vi "Parameter Set Write Single.vi"() -> ()   [LabVIEW 2023, in "Cycler.lvclass"]
uses:
  Cycler.lvclass
  Low Level Capabilities/Parameter Set/Parameter Set.lvclass
panel:
  in  "Channel Index":i32
  in  "Parameter Set STS":i32
  out "error out":errorcluster
  in  "error in":errorcluster
  out "Cycler out":refnum<class "Cycler.lvclass">
  in  "Cycler in":refnum<class "Cycler.lvclass">
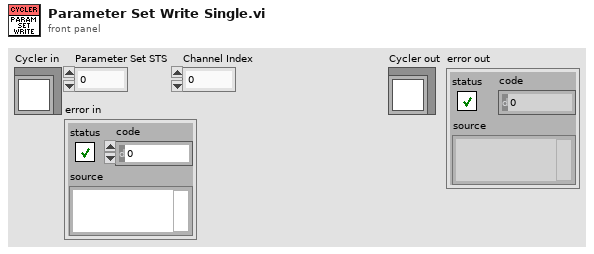
[diagram p1: front panel]
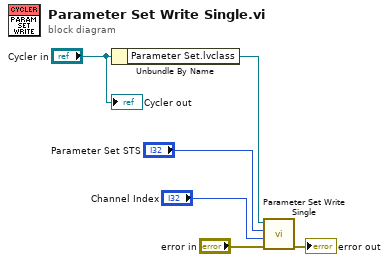
[diagram p0: block diagram]
diagram:
  n1 = Unbundle By Name("Cycler in") -> ("Parameter Set.lvclass"=w5:refnum<class "Parameter Set.lvclass">)
  n2 = call-dynamic "Parameter Set Write Single.vi"("error in"="error in", "Channel Index"="Channel Index", "Parameter Set STS"="Parameter Set STS", "Parameter Set in"=w5) -> ("error out"=→"error out":errorcluster)  [unwired: 6 in, 1 out]
  "Cycler out" <- "Cycler in"
